vi "Unflatten.vi"(8 "error in (no error)":errorcluster, 11 "Microwave Freq Scan in":refnum<class "Microwave Freq Scan.lvclass">) -> (0 "error out":errorcluster, 3 "Microwave Freq Scan out":refnum<class "Microwave Freq Scan.lvclass">)   [LabVIEW 2017, in "Microwave Freq Scan.lvclass"]
uses:
  Microwave Freq Scan.lvclass
  Microwave Freq Scan.lvclass/Microwave Freq Scan.ctl
  Global/File Locations.vi
  Scanner/Scanner.lvclass
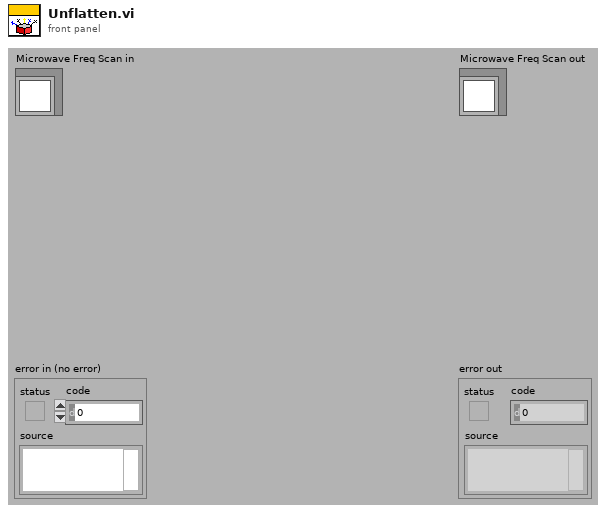
[diagram p1: front panel]
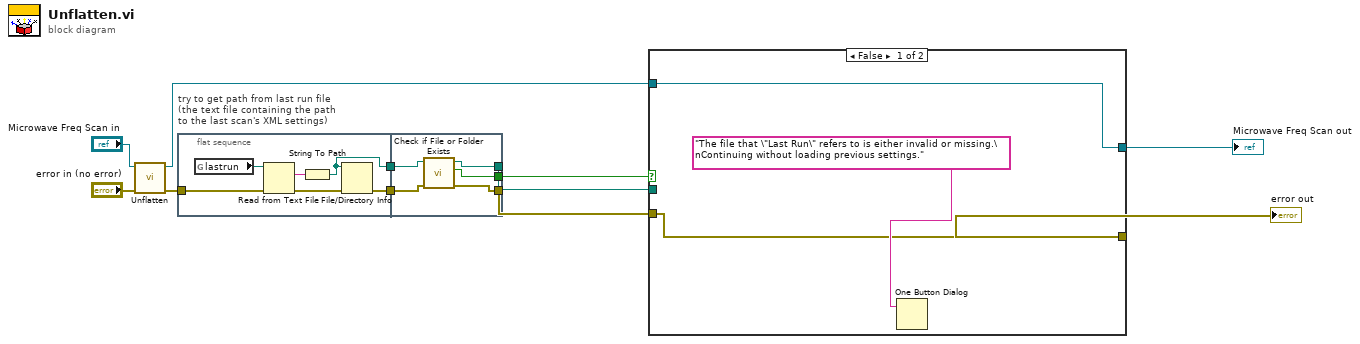
[diagram p0: block diagram]
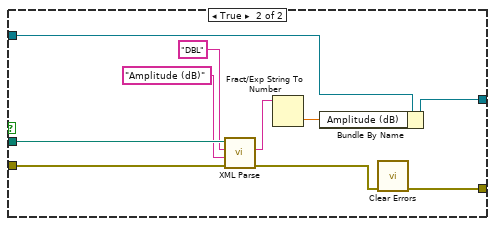
[diagram p2: hidden frame]
diagram:
  n1 = call-parent "Unflatten.vi"("error in (no error)"="error in (no error)", "Scanner in"="Microwave Freq Scan in") -> ("error out"=w7:errorcluster, "Scanner out"=w11:refnum<class "Microwave Freq Scan.lvclass">)  [unwired: 8 in]
  n2 = flat-sequence "try to get path from last run file\n(the text file containing the path\nto the last scan's XML settings)" {
    tunnel: w7 -> [w12]
    tunnel: [w17] -> w3
    tunnel: [w13] -> w2
    tunnel: [w19] -> w5
    tunnel: [w21] -> w6
    tunnel: w3 -> [w22]
    tunnel: w2 -> [w18]
    tunnel: [w20] -> w1
    frame #0 {
      n3 = global read "File Locations.vi" "lastrun"() -> (w15:path)
      n4 = Read from Text File(file (use dialog)=w15, error in=w12) -> (text=w16:string, error out=w14:errorcluster)  [unwired: 4 out]
      n5 = String To Path(string=w16) -> (path=w17:path)
      n6 = File/Directory Info(path=w17, error in=w14) -> (error out=w13:errorcluster)  [unwired: 6 out]
    }
    frame #1 {
      n7 = call <vilib>:"Check if File or Folder Exists.vi"("error in (no error)"=w18, "path"=w22) -> ("error out"=w19:errorcluster, "file or folder exists?"=w20:bool, "dup path"=w21:path)  [unwired: 7 in]
    }
  }
  n8 = case shown="False" w1 {
    tunnel: w11 -> [w23 w35]
    tunnel: [w23 w34] -> w8
    tunnel: w6 -> [_ w33]
    tunnel: w5 -> [w24 w32]
    tunnel: [w24 w26] -> w4
    frame False {
      n9 = One Button Dialog(message="The file that \"Last Run\" refers to is either invalid or missing.\nContinuing without loading previous settings.") -> ()  [unwired: 1 in, 1 out]
    }
    frame True {
      n10 = call "XML Parse.vi"("error in (no error)"=w32, "Name String"="Amplitude (dB)", "Type String"="DBL", "Path"=w33) -> ("error out"=w31:errorcluster, "String Out"=w27:string)  [unwired: 6 in]
      n11 = Fract/Exp String To Number(string=w27) -> (number=w28:dbl)  [unwired: 3 in, 1 out]
      n12 = Bundle By Name(cluster=w35, "Amplitude (dB)"=w28) -> (w34:refnum<class "Microwave Freq Scan.lvclass">)
      n13 = call <vilib>:"Clear Errors.vi"("error in (no error)"=w31) -> ("error out"=w26:errorcluster)  [unwired: 5 in, 1 out]
    }
  }
  "error out" <- w4
  "Microwave Freq Scan out" <- w8
